vi "ProcessPAQsample.vi"(8 "error in (no error)":errorcluster, 10 "PAQdatagram IN":T1 {"data" format="%.2f"; "status" format="%08x"}, 11 "AVPP in":refnum<class "AVPP.lvclass">) -> (0 "error out":errorcluster, 3 "AVPP out":refnum<class "AVPP.lvclass">)   [LabVIEW 2014, in "AVPP.lvclass"]
doc: "AVPP process request for an PAQ sample (array of TAGs containing one sample for each TAG)"
uses:
  AVPP.lvclass
  HISW/controls/typedef_PAQdatagram.ctl
  FAMM/controls/typedef_Level.ctl
  FAMM/controls/typedef_AverageAction.ctl
  FAMM/FAMM.lvclass
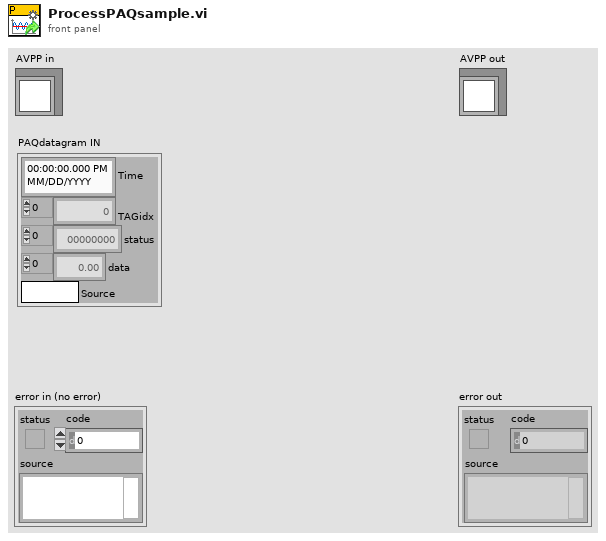
[diagram p1: front panel]
types:
  T1 = typedef "typedef_PAQdatagram.ctl" = cluster{"Time":timestamp, "TAGidx":i32[], "status":u32[], "data":dbl[], "Source":string}
  T2 = typedef "typedef_AverageAction.ctl" = cluster{"Level":T3, "HigherLevel":bool, "prev_pnt":i32, "last_pnt":i32}
  T3 = typedef "typedef_Level.ctl" = enum16{"L0_PAQ_10mil", "L0_PAQ_100mil", "L1_PAQ_100mil", "L2_PAQ_1sec", "L3_PAQ_10sec", "L4_PAQ_1min", "L5_PAQ_10min", "L6_PAQ_2hr", "L7_PAQ_1day", "L8_PAQ_1wk", "L1_PAQ_1sec", "L2_PAQ_10sec", "L3_PAQ_1min", "L4_PAQ_10min", "L5_PAQ_2hr", "L6_PAQ_1day", "L7_PAQ_1wk", "L0_PAQ_1sec", "L1_PAQ_10sec", "L2_PAQ_1min", "L3_PAQ_10min", "L4_PAQ_2hr", "L5_PAQ_1day", "L6_PAQ_1wk", "L0_PAQ_10sec", "L1_PAQ_1min", "L2_PAQ_10min", "L3_PAQ_2hr", "L4_PAQ_1day", "L5_PAQ_1wk"}
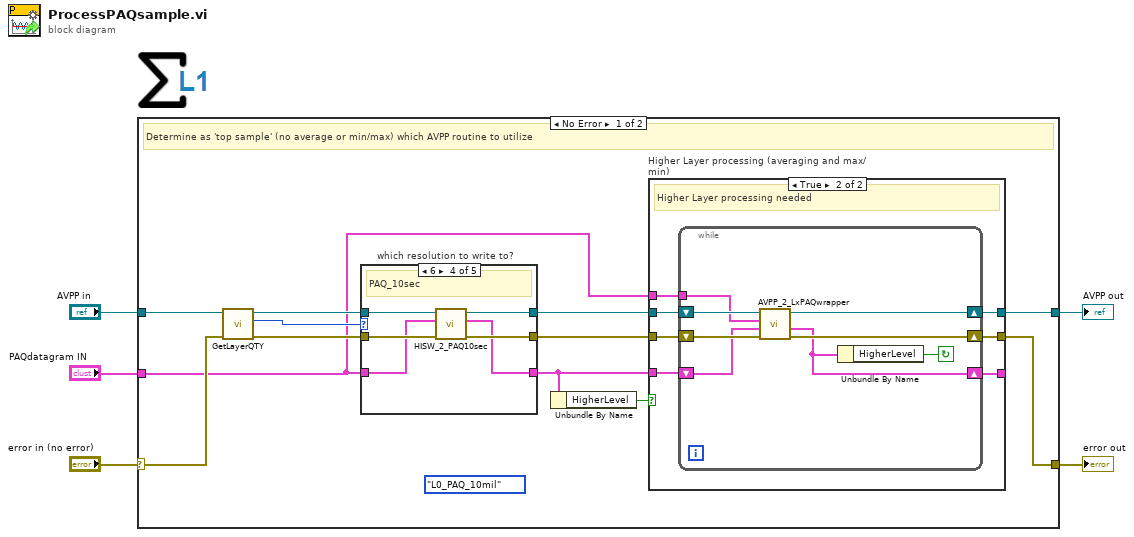
[diagram p0: block diagram]
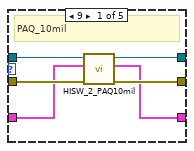
[diagram p3: hidden frame]
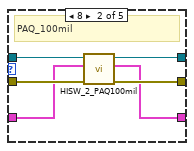
[diagram p4: hidden frame]
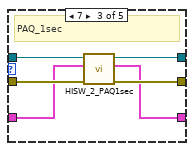
[diagram p5: hidden frame]
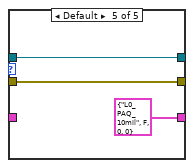
[diagram p6: hidden frame]
diagram:
  n1 = case "PAQ write : Abstraction level AB1 (in AVPP)" shown="No Error" "error in (no error)" {
    selector: "error in (no error)" -> [w16 w64]
    tunnel: [w9 w64] -> w4
    tunnel: [w10 w63] -> w2
    tunnel: "AVPP in" -> [w17 w63]
    tunnel: "PAQdatagram IN" -> [w8 _]
    frame No Error {
      (unwired) typedef_Level."L0_PAQ_10mil" ("Level")
      # "Determine as 'top sample' (no average or min/max) which AVPP routine to utilize"
      n2 = call "GetLayerQTY.vi"("error in (no error)"=w16, "FAMM in"=w17) -> ("error out"=w13:errorcluster, "FAMM_PAQ_Layers"=w15:i32, "FAMM out"=w14:refnum<class "AVPP.lvclass">)  [unwired: 6 in, 1 out]
      n3 = case "which resolution to write to?" shown="6" w15 {
        tunnel: w8 -> [w37 w43 w49 w55 _]
        tunnel: w14 -> [w41 w47 w53 w59 w62]
        tunnel: w13 -> [w40 w46 w52 w58 w61]
        tunnel: [w38 w44 w50 w56 w62] -> w12
        tunnel: [w39 w45 w51 w57 w61] -> w11
        tunnel: [w36 w42 w48 w54 T2 {"Level"=enum."L0_PAQ_10mil", "HigherLevel"=FALSE, "prev_pnt"=0, "last_pnt"=0} ("AverageAction")] -> w6
        frame 9 {
          # "PAQ_10mil"
          n4 = call "HISW_2_PAQ10mil.vi"("error in (no error)"=w40, "PAQdatagram IN"=w37, "AVPP in"=w41) -> ("error out"=w39:errorcluster, "Next_Level"=w36:T2, "AVPP out"=w38:refnum<class "AVPP.lvclass">)  [unwired: 6 in]
        }
        frame 8 {
          # "PAQ_100mil"
          n5 = call "HISW_2_PAQ100mil.vi"("error in (no error)"=w46, "PAQdatagram IN"=w43, "AVPP in"=w47) -> ("error out"=w45:errorcluster, "Next_Level"=w42:T2, "AVPP out"=w44:refnum<class "AVPP.lvclass">)  [unwired: 6 in]
        }
        frame 7 {
          # "PAQ_1sec"
          n6 = call "HISW_2_PAQ1sec.vi"("error in (no error)"=w52, "PAQdatagram IN"=w49, "AVPP in"=w53) -> ("error out"=w51:errorcluster, "Next_Level"=w48:T2, "AVPP out"=w50:refnum<class "AVPP.lvclass">)  [unwired: 6 in]
        }
        frame 6 {
          # "PAQ_10sec"
          n7 = call "HISW_2_PAQ10sec.vi"("error in (no error)"=w58, "PAQdatagram IN"=w55, "AVPP in"=w59) -> ("error out"=w57:errorcluster, "Next_Level"=w54:T2, "AVPP out"=w56:refnum<class "AVPP.lvclass">)  [unwired: 6 in]
        }
        frame Default {
        }
      }
      n8 = Unbundle By Name(w6) -> ("HigherLevel"=w7:bool)
      n9 = case "Higher Layer processing (averaging and max/min)" shown="True" w7 {
        tunnel: w12 -> [w20 w26]
        tunnel: w11 -> [w19 w27]
        tunnel: w6 -> [w18 w23]
        tunnel: [w20 w25] -> w10
        tunnel: [w19 w24] -> w9
        tunnel: w8 -> [_ w22]
        tunnel: [w18 w21] -> _
        frame False {
          # "no averaging needed"
        }
        frame True {
          # "Higher Layer processing needed"
          n10 = while {
            shift-right: [w34] -> w25
            shift-left: w26 -> [w35]
            shift-right: [w32] -> w24
            shift-left: w27 -> [w33]
            shift-right: [w30] -> w21
            shift-left: w23 -> [w28]
            tunnel: w22 -> [w29]
            stop <- w31 continue-if-true
            n11 = call "AVPP_2_LxPAQwrapper.vi"("error in (no error)"=w33, "AverageAction IN"=w28, "PAQdatagram IN"=w29, "AVPP in"=w35) -> ("error out"=w32:errorcluster, "Next_Level"=w30:T2, "AVPP out"=w34:refnum<class "AVPP.lvclass">)  [unwired: 5 in]
            n12 = Unbundle By Name(w30) -> ("HigherLevel"=w31:bool)
          }
        }
      }
    }
    frame Error {
    }
  }
  "error out" <- w4
  "AVPP out" <- w2
